vi "Reset.vi"(8 "error in (no error)":errorcluster, 11 "NISTSimulation in":refnum<class "Simulation.lvclass">) -> (0 "error out":errorcluster, 3 "NISTSimulation out":refnum<class "Simulation.lvclass">)   [LabVIEW 2014, in "SamplerPlugins.lvlib" / "Simulation.lvclass"]
uses:
  Simulation.lvclass
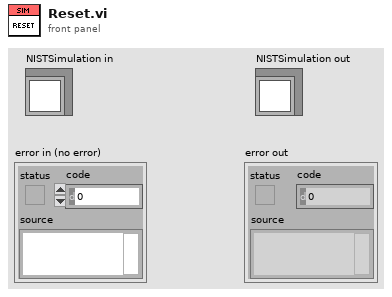
[diagram p1: front panel]
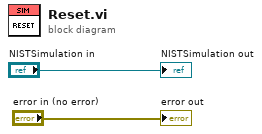
[diagram p0: block diagram]
diagram:
  "error out" <- "error in (no error)"
  "NISTSimulation out" <- "NISTSimulation in"
